vi "rethinkdb_json_elements_reorder.vi"(7 "type elements":variant[](array[variant]), 8 "error in (no error)":errorcluster, 9 "allow missing?":bool, 11 "json elements":variant[](array[variant])) -> (0 "error out":errorcluster, 1 "complete match?":bool, 3 "reordered json elements":variant[](array[variant]))   [LabVIEW 2017]
uses:
  <vilib>/Utility/Data Type/NI_Data Type.lvlib
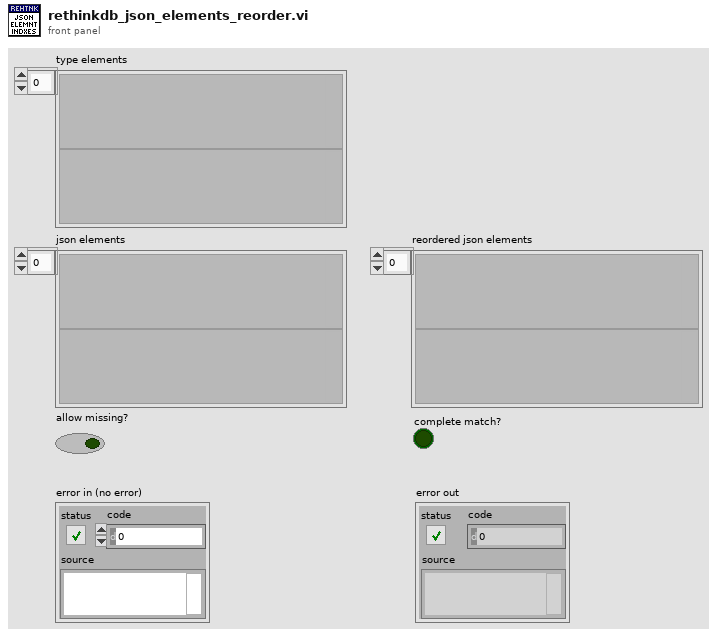
[diagram p1: front panel]
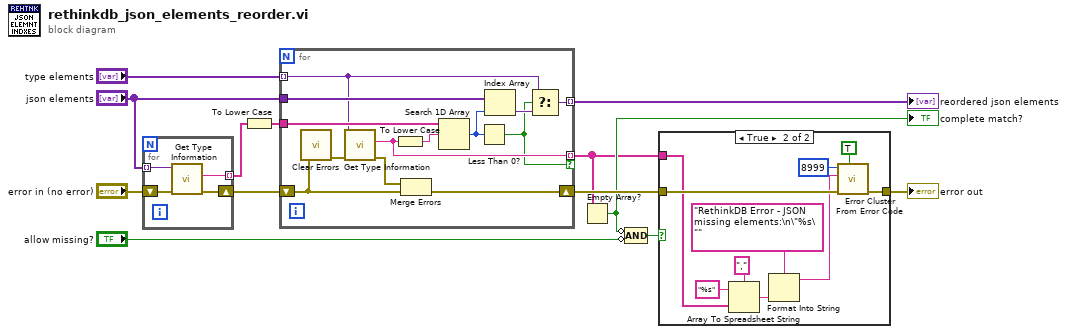
[diagram p0: block diagram]
diagram:
  n1 = for {
    shift-right: [w15] -> w9
    shift-left: "error in (no error)" -> [w17]
    tunnel: "json elements" -> [w16] mode=indexing
    tunnel: [w14] -> w13 mode=indexing
    n2 = call <vilib>:"Get Type Information.vi"("error in (no error)"=w17, "Variant"=w16) -> ("error out"=w15:errorcluster, "Name"=w14:string)  [unwired: 5 in, 3 out]
  }
  n3 = To Lower Case(string=w13) -> (all lower case string=w12:string[])
  n4 = for {
    shift-right: [w20] -> w5
    shift-left: w9 -> [w19]
    tunnel: "type elements" -> [w25] mode=indexing
    tunnel: w12 -> [w29]
    tunnel: "json elements" -> [w28]
    tunnel: [w26] -> w7 mode=indexing
    tunnel: [w22] -> w1 mode=indexing if=w18
    n5 = call <vilib>:"Clear Errors.vi"("error in (no error)"=w19) -> ("error out"=w21:errorcluster)  [unwired: 5 in, 1 out]
    n6 = call <vilib>:"Get Type Information.vi"("error in (no error)"=w21, "Variant"=w25) -> ("error out"=w23:errorcluster, "Name"=w22:string)  [unwired: 5 in, 3 out]
    n7 = To Lower Case(string=w22) -> (all lower case string=w30:string)
    n8 = Merge Errors(w23, w19) -> (w20:errorcluster)
    n9 = Search 1D Array(1D array=w29, element=w30) -> (index of element=w27:i32)  [unwired: 1 in]
    n10 = Less Than 0?(x=w27) -> (x < 0?=w18:bool)
    n11 = Index Array(array=w28, index=w27) -> (element=w24:variant)
    n12 = Select(t=w25, s=w18, f=w24) -> (s? t:f=w26:variant)
  }
  "reordered json elements" <- w7
  n13 = Empty Array?(array=w1) -> (empty?=w2:bool)
  "complete match?" <- w2
  n14 = Compound Arithmetic op=AND(invert w2, invert "allow missing?") -> (w3:bool)
  n15 = case shown="True" w3 {
    tunnel: w5 -> [w31 w41]
    tunnel: [w31 w40] -> w4
    tunnel: w1 -> [_ w35]
    frame False {
    }
    frame True {
      n16 = Array To Spreadsheet String(delimiter (Tab)=",", array=w35, 3:"%s" ("format string")) -> (spreadsheet string=w32:string)
      n17 = Format Into String(format string="RethinkDB Error - JSON missing elements:\n\"%s\"" ("error message (\"\")"), w32) -> (resulting string=w36:string)  [unwired: 2 in, 1 out]
      n18 = call <vilib>:"Error Cluster From Error Code.vi"("show call chain? (False)"=TRUE, "error in (no error)"=w41, "error message (\"\")"=w36, "error code (0)"=8999) -> ("error out"=w40:errorcluster)  [unwired: 5 in]
    }
  }
  "error out" <- w4
